vi "UniversalTimestampInSeconds.vi"() -> (0 "Difference that should match C++ timestamp":dbl format="%#_14g", 1 "current time":timestamp)   [LabVIEW 2010]
uses:
  <vilib>/Utility/miscctls.llb/LVDateTimeRec.ctl
panel:
  out "Number of Seconds from 1904 to Jan 1 1972":dbl format="%#_14g"
  out "time stamp 2":timestamp
  out "Total Number of seconds from 1904 to now":dbl format="%#_14g"
  out "date time rec":T1
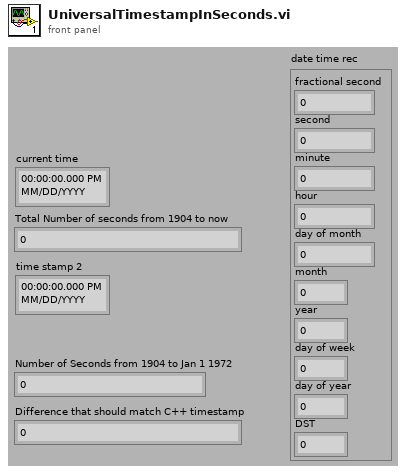
[diagram p1: front panel]
types:
  T1 = typedef "LVDateTimeRec.ctl" = cluster{"fractional second":dbl, "second":i32, "minute":i32, "hour":i32, "day of month":i32, "month":i32, "year":i32, "day of week":i32, "day of year":i32, "DST":i32}
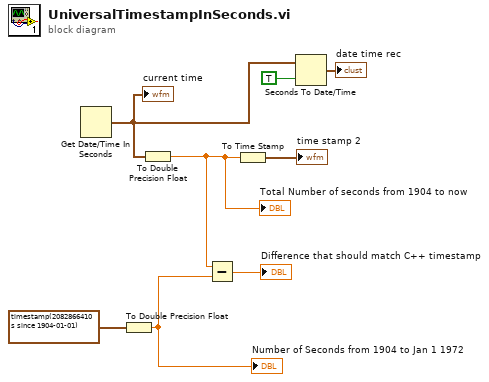
[diagram p0: block diagram]
diagram:
  n1 = Get Date/Time In Seconds() -> (seconds since 1Jan1904=w6:timestamp)
  "current time" <- w6
  n2 = To Double Precision Float(number=timestamp(2082866410 s since 1904-01-01)) -> (double precision float=w3:dbl)
  "Number of Seconds from 1904 to Jan 1 1972" <- w3
  n3 = To Double Precision Float(number=w6) -> (double precision float=w2:dbl)
  "Total Number of seconds from 1904 to now" <- w2
  n4 = Subtract(x=w2, y=w3) -> (x-y=→"Difference that should match C++ timestamp":dbl)
  n5 = To Time Stamp(1:w2) -> (0:→"time stamp 2":timestamp)
  n6 = Seconds To Date/Time(time stamp (now)=w6, to UTC (F)=TRUE) -> (date time rec=→"date time rec":T1)
